vi "launch.vi"(8 "error in (no error)":errorcluster, 11 "CameraControlViewer in":refnum<class "CameraControlViewer.lvclass">) -> (0 "error out":errorcluster, 3 "CameraControlViewer out":refnum<class "CameraControlViewer.lvclass">)   [LabVIEW 2009, in "Views.lvlib" / "Camera.lvlib" / "CameraControlViewer.lvclass"]
uses:
  CameraControlViewer.lvclass
  Tools/Filing/FileSystem/FileSystem.lvclass
  CameraControlViewer.lvclass/CameraControlViewer.ctl
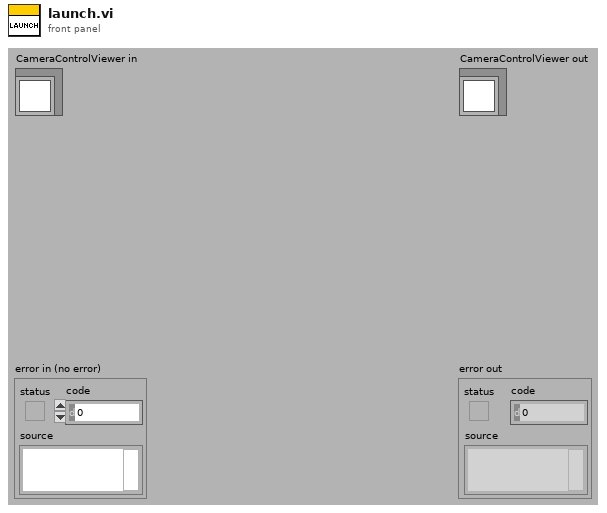
[diagram p1: front panel]
types:
  T1 = enum32{"Invalid", "Standard", "Closed", "Hidden", "Minimized", "Maximized"}
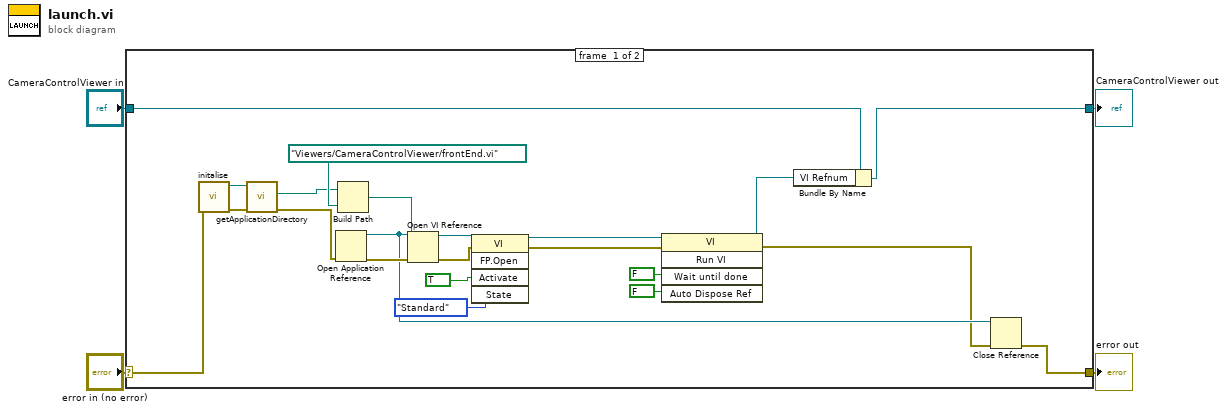
[diagram p0: block diagram]
diagram:
  n1 = case shown="No Error" "error in (no error)" {
    selector: "error in (no error)" -> [w11 w28]
    tunnel: [w5 w28] -> w3
    tunnel: [w6 w27] -> w1
    tunnel: "CameraControlViewer in" -> [w7 w27]
    frame #0 {
      n2 = call "initalise.vi"("error in (no error)"=w11) -> ("error out"=w16:errorcluster, "FileSystem out"=w17:refnum<class "FileSystem.lvclass">)  [unwired: 9 in]
      n3 = call-dynamic "getApplicationDirectory.vi"("error in (no error)"=w16, "FileSystem.lvclass in"=w17) -> ("error out"=w12:errorcluster, "ApplicationDirectory"=w14:path)  [unwired: 7 in, 1 out]
      n4 = Open Application Reference(8:w12) -> (0:w24:errorcluster, 3:w23:refnum<vi>)  [unwired: 3 in]
      n5 = Build Path(base path=w14, name or relative path=path "Viewers/CameraControlViewer/frontEnd.vi" ("vi path")) -> (appended path=w13:path)
      n6 = Open VI Reference(application reference (local)=w23, vi path=w13, error in (no error)=w24) -> (vi reference=w21:refnum<vi>, error out=w20:errorcluster)  [unwired: 3 in]
      n7 = invoke class="VI" method="FP.Open"(reference=w21, error in=w20, "Activate"=TRUE, "State"=T1."Standard") -> (reference out=w10:refnum<vi>, error out=w9:errorcluster)  [unwired: 1 in, 3 out]
      n8 = invoke class="VI" method="Run VI"(reference=w10, error in=w9, "Wait until done"=FALSE, "Auto Dispose Ref"=FALSE) -> (reference out=w8:refnum<vi>, error out=w22:errorcluster)  [unwired: 1 in, 3 out]
      n9 = Bundle By Name(cluster=w7, "VI Refnum"=w8) -> (w6:refnum<class "CameraControlViewer.lvclass">)
      n10 = Close Reference(reference=w23, error in (no error)=w22) -> (error out=w5:errorcluster)
    }
    frame #1 {
    }
  }
  "error out" <- w3
  "CameraControlViewer out" <- w1
